vi "运维调试_总磷总氮.vi"() -> ()   [LabVIEW 2016, in "斯坦道总磷总氮.lvlib"]
uses:
  <vilib>/Utility/miscctls.llb/LVPointTypeDef.ctl
  <vilib>/Plasmionique/MB Master/MB_Master/MB_Master.lvclass
  <vilib>/ptbypt/NI_PtbyPt.lvlib
panel:
  out "步骤":u16
  out "seconds since 1Jan1904 2":timestamp
  out "seconds since 1Jan1904":timestamp
  in  "周期设置":bool
  in  "流程操作":bool
  out "消解压力":sgl format="%#.2f kPa"
  out "权限等级":string
  out "总步数":i32
  out "滑动杆":dbl(slide) caption="测试进度" scale=0.0..100.0
  out "试剂余量显示":sgl[][](graph)
  in  "仪器校准":bool
  in  "参数查询":bool
  out "简易步骤名称":string
  in  "温度曲线":bool
  in  "试剂余量":bool
  in  "灯值调整":bool
  out "固件版本号":string
  out "模块版本号":string
  out "注射器温度":sgl format="%#.2f ℃"
  out "消解温度":sgl format="%#.2f ℃"
  out "ADC":sgl
  out "F3":sgl format="%#.6f"
  out "F2":sgl format="%#.6f"
  out "F1":sgl format="%#.6f"
  out "F0":sgl format="%#.6f"
  out "运行状态":T1 {"数据时间:" format="%<%y/%m/%d %H:%M:%S>T"; "仪器时间:" format="%<%y/%m/%d %H:%M:%S>T"}
  in  "单选按钮":T2=enum."总氮"
  in  "布尔":bool
  in  "外设固件":bool
  out "字符串 2":string
  in  "数组":string[](array[string])
  in  "返回":bool
  in  "参数设置":bool
  out "集成报警信息":string
  in  "停止":bool
  in  "手动启动":bool
  in  "调试":bool
  out "多列列表框":i32(listbox)
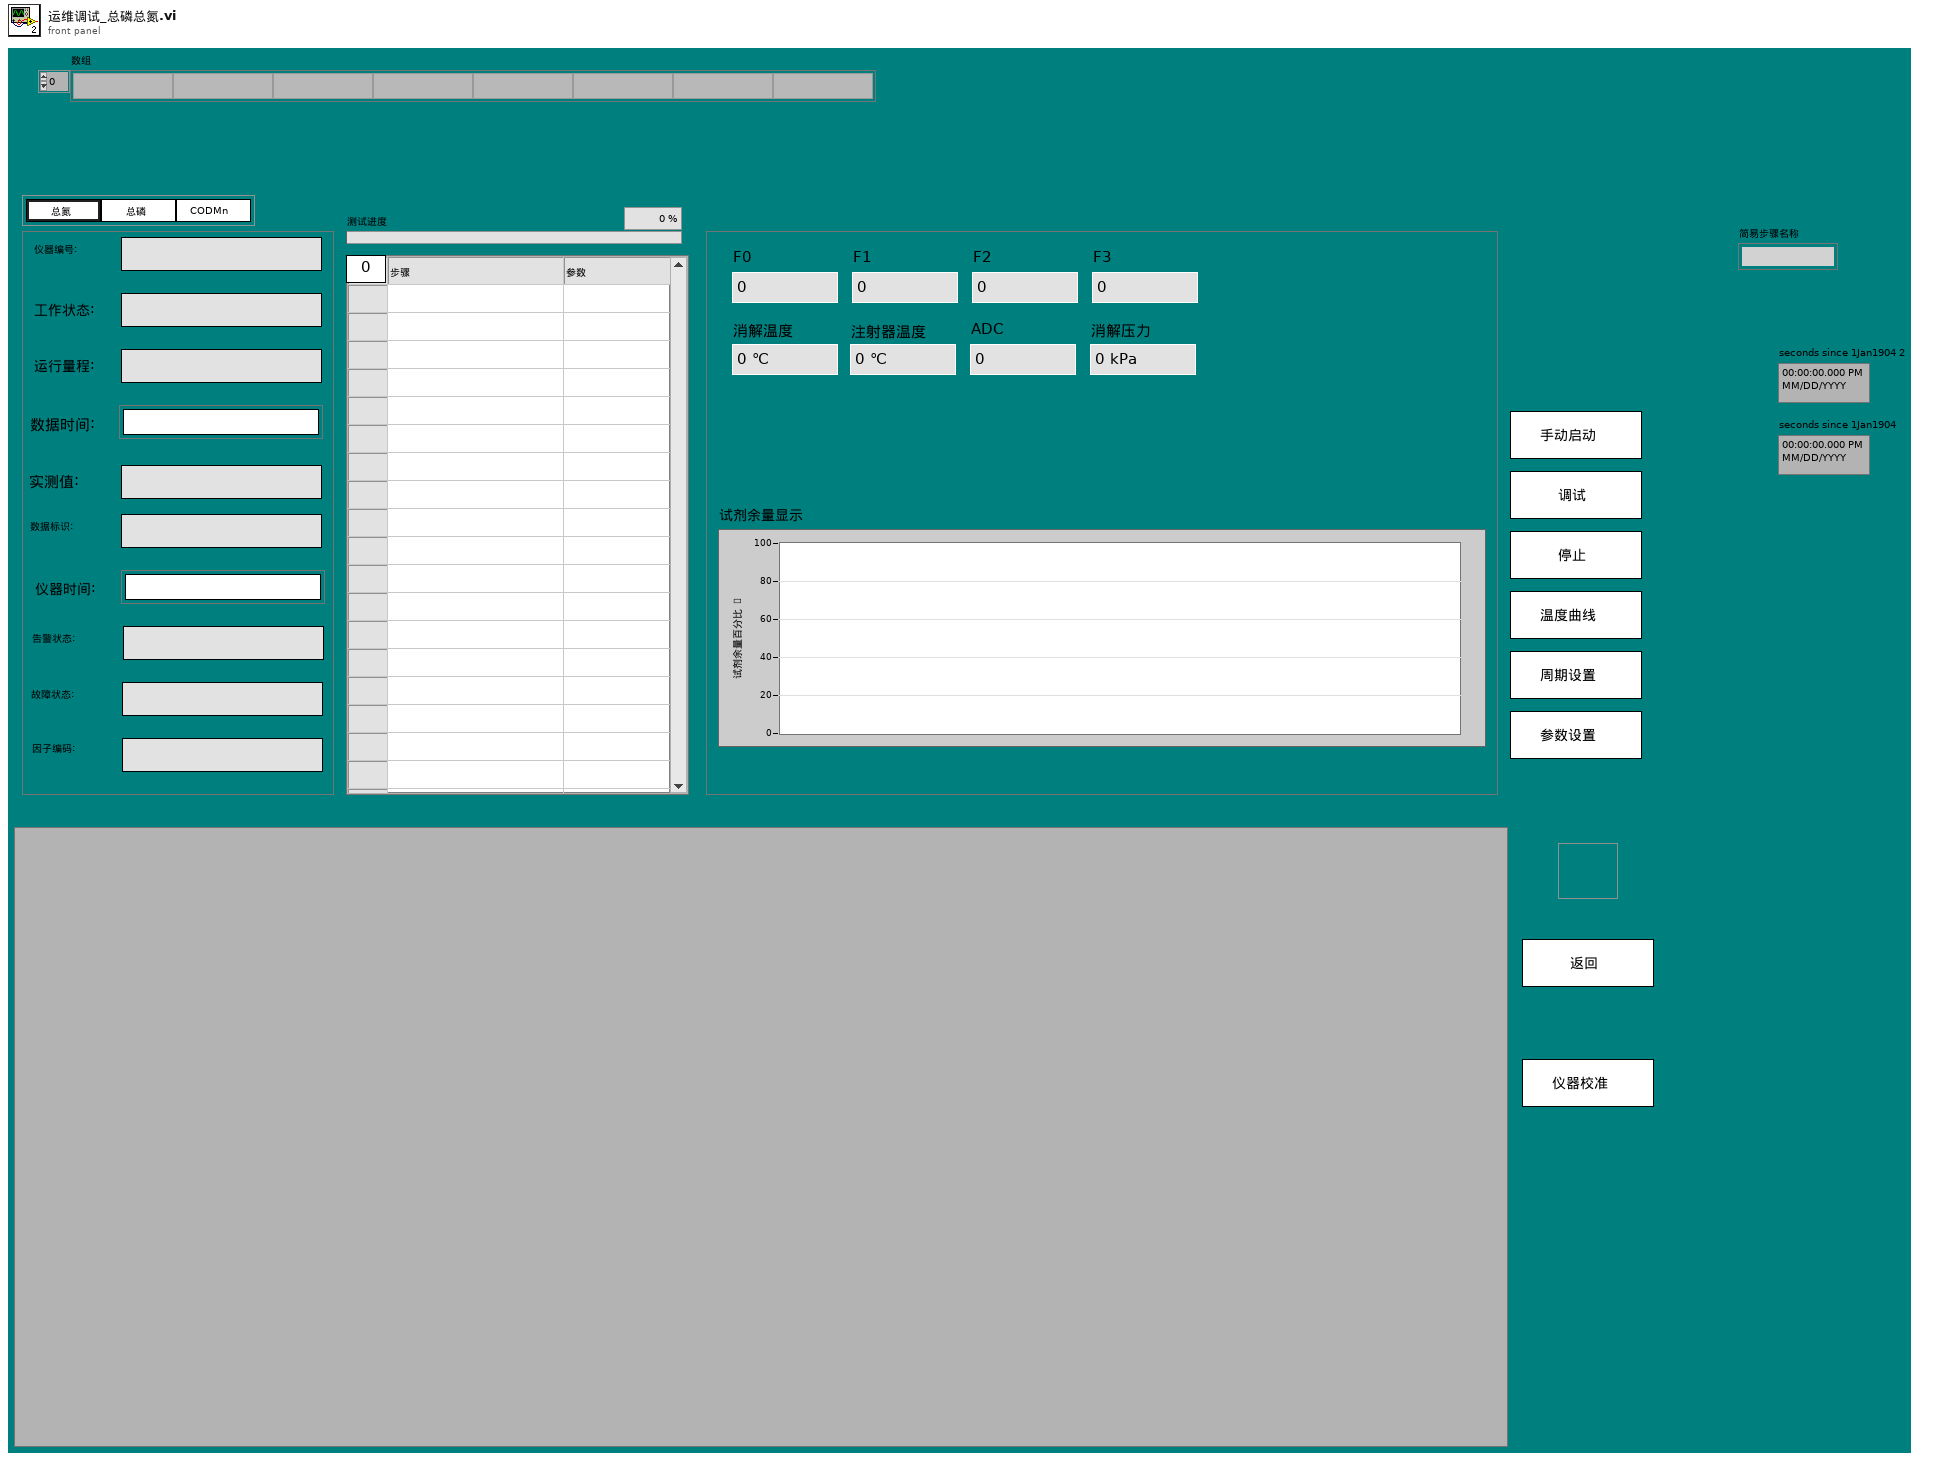
[diagram p1: front panel]
types:
  T1 = cluster{"仪器编号:":string, "工作状态:":string, "运行量程: ":string, "数据时间:":timestamp, "实测值:":string, "数据标识: ":string, "仪器时间:":timestamp, "告警状态: ":string, "故障状态:  ":string, "因子编码:":string}
  T2 = typedef "斯坦道总磷总氮.lvlib/启动参数显示控件.ctl" = enum32{"COD", "氨氮", "总氮", "总磷", "磷酸盐", "硝氮", "亚硝氮", "硅酸盐", "硫化物", "氟化物", "CODMn"}
  T3 = typedef "LVPointTypeDef.ctl" = cluster{"Horizontal":i16, "Vertical":i16}
  T4 = cluster{"系统时间":timestamp, "工作状态":u16, "测量模式":enum16{"待机", "连续模式", "周期模式", "定点模式", "受控模式", "手动模式"}, "告警代码":u16, "故障代码":u16, "日志代码":u16, "软件版本":u16, "F0":sgl, "F1":sgl, "F2":sgl, "F3":sgl, "T":sgl, "H":sgl, "id":u16, "flowid":u16, "量程":u16, "总磷控温温度1":sgl, "营养盐控温温度2":sgl, "ADC":sgl, "结果值":sgl, "运行时间":u16, "步骤详情":string, "步骤流程":string}
  T5 = cluster{"Major":u16, "Minor":u16, "Fix":u16, "Build":u16}
  T6 = typedef "LVStringsAndValuesArrayTypeDef_U16.ctl" = cluster{"String":string, "Value":u16}[]
  T7 = cluster{"因子编码":u32, "单位":u16, "标样参考值":sgl, "水样数据时间":timestamp, "水样实测值":sgl, "水样数据标识":string, "标样数据时间":timestamp, "标样实测值":sgl, "标样数据标识":string, "空白数据时间":timestamp, "空白实测值":sgl, "空白数据标识":string, "零点核查数据时间":timestamp, "零点核查实测值":sgl, "零点核查数据标识":string, "跨度核查数据时间":timestamp, "跨度核查实测值":sgl, "跨度核查数据标识":string, "加标回收数据时间":timestamp, "加标回收实测值":sgl, "加标回收数据标识":string, "平行样数据时间":timestamp, "平行样实测值":sgl, "平行样数据标识":string, "F0":sgl, "F1":sgl, "F2":sgl, "F3":sgl, "F4":sgl, "F5":sgl, "F6":sgl, "F7":sgl, "温度":sgl, "湿度":sgl, "X值":sgl, "fidrange":u16, "X1值":sgl}[]
  T8 = typedef "SingleStepTestV3.lvlib/SingleStepTestV3.lvclass/仪器版本.ctl" = enum16{"V3.1版", "V4版", "V3版", "V4.2版"}
  T9 = cluster{"因子编码":u32, "单位":u16, "标样参考值":sgl, "水样数据时间":timestamp, "水样实测值":sgl, "水样数据标识":string, "标样数据时间":timestamp, "标样实测值":sgl, "标样数据标识":string, "空白数据时间":timestamp, "空白实测值":sgl, "空白数据标识":string, "零点核查数据时间":timestamp, "零点核查实测值":sgl, "零点核查数据标识":string, "跨度核查数据时间":timestamp, "跨度核查实测值":sgl, "跨度核查数据标识":string, "加标回收数据时间":timestamp, "加标回收实测值":sgl, "加标回收数据标识":string, "平行样数据时间":timestamp, "平行样实测值":sgl, "平行样数据标识":string, "F0":sgl, "F1":sgl, "F2":sgl, "F3":sgl, "F4":sgl, "F5":sgl, "F6":sgl, "F7":sgl, "温度":sgl, "湿度":sgl, "X值":sgl, "fidrange":u16, "X1值":sgl}
  T10 = typedef "Alarm interface.lvlib/报警短信语音交互.ctl" = cluster{"参数":string, "元器件":string, "故障现象":string, "code":string, "platform_alarm_code":string, "solutionList":cluster{"reason":string, "solution":string}[], "是否上报":string}
  T11 = typedef "TimingControl.lvlib/TimingControl.lvclass/国标控制命令.ctl" = enum16{"启动测量", "标样核查", "零点核查", "跨度核查", "空白测试", "平行样测试", "加标回收", "空白校准", "标样校准", "初始化（清洗）", "停止测试", "仪器重启", "校时", "模式设置", "测量间隔设置"}
  T12 = typedef "TimingControl.lvlib/TimingControl.lvclass/测量参数.ctl" = u16
  T13 = enum32{"Bad", "Idle", "Run top level", "Running"}
  T14 = cluster{"时间标识":timestamp, "设备":string, "日志信息":string, "流程参数":string}
  T15 = typedef "LVRowAndColumnUnsignedTypeDef.ctl" = cluster{"Row":u32, "Column":u32}
  T16 = typedef "操作日志字段定义.ctl" = cluster{"时间":timestamp, "参数":string, "日志信息":string, "流程参数":string}
  T17 = cluster{"站号":u16, "量程切换":enum32{"H", "L", "AUTO"}, "控制命令":enum16{"启动测量", "标样核查", "零点核查", "跨度核查", "空白测试", "平行样测试", "加标回收", "空白校准", "标样校准", "初始化（清洗）", "停止测试", "仪器重启", "校时", "模式设置", "测量间隔设置"}, "模式设置":enum16{"待机", "连续模式", "周期模式", "定点模式", "受控模式", "手动模式"}, "测量间隔":u16}
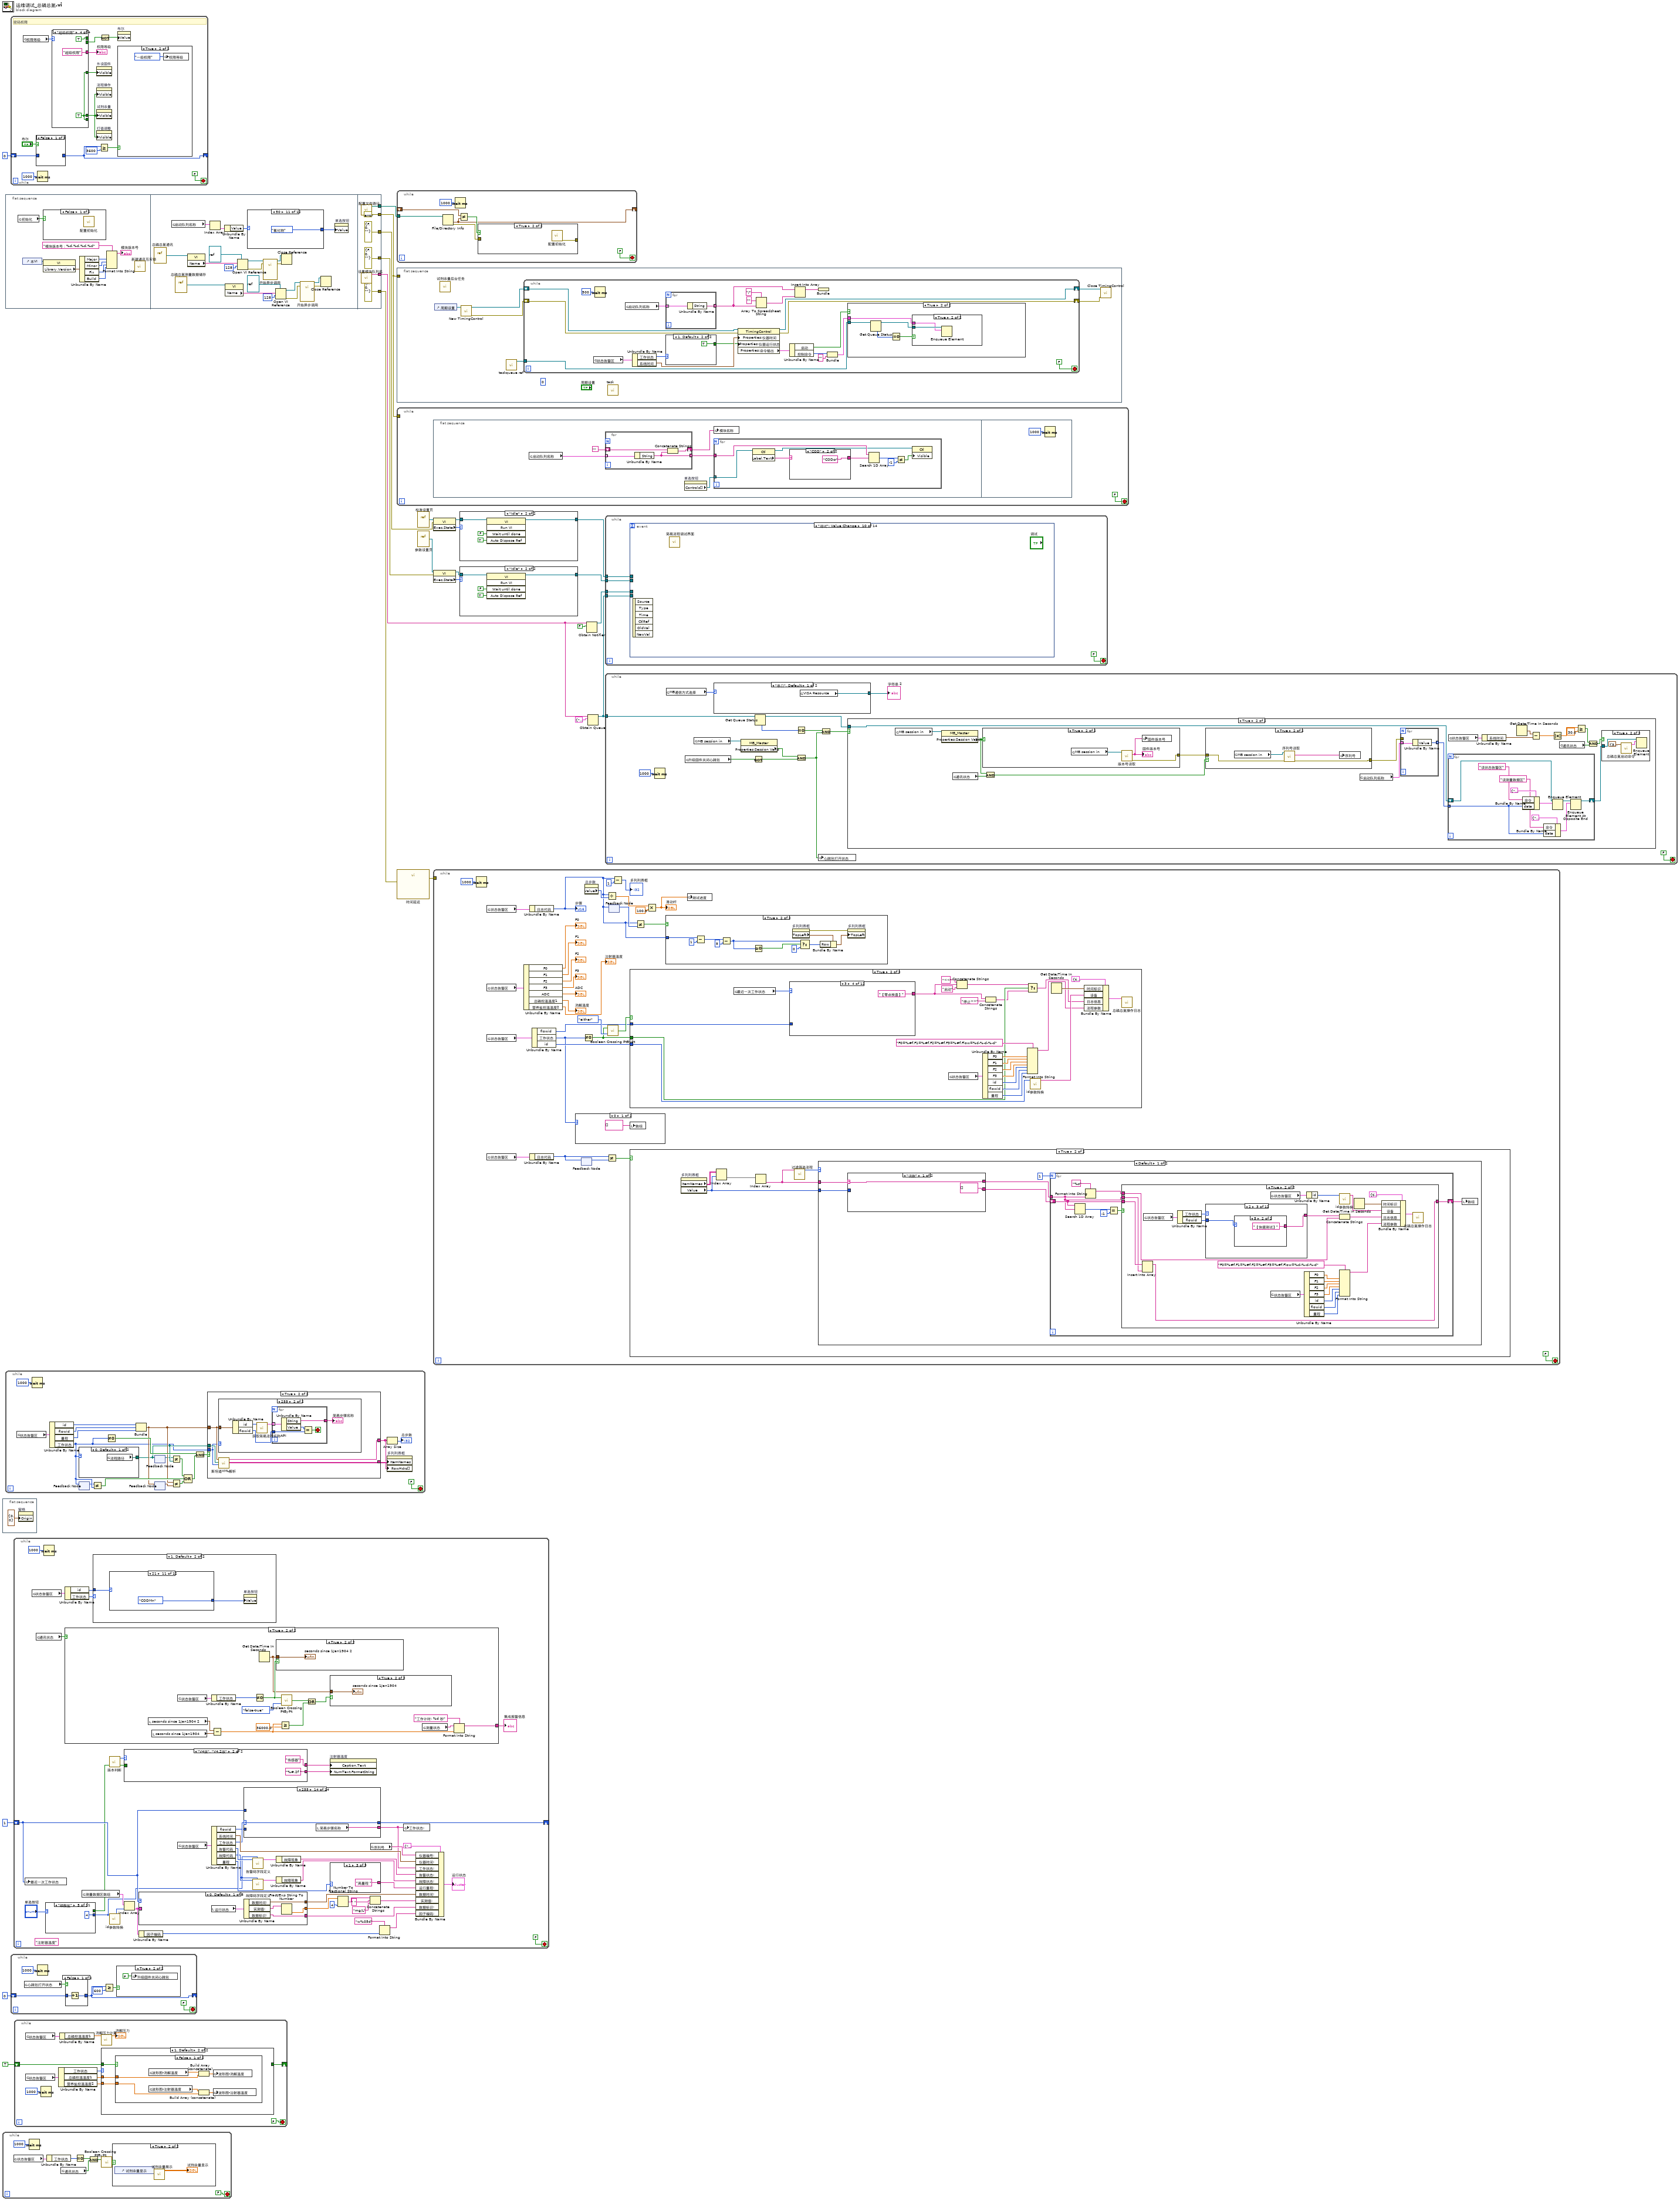
[diagram p0: block diagram]
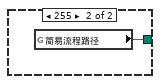
[diagram p2: hidden frame]
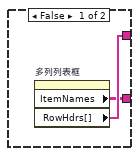
[diagram p3: hidden frame]
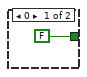
[diagram p7: hidden frame]
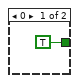
[diagram p14: hidden frame]
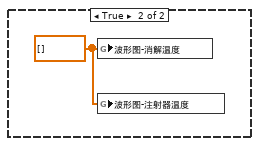
[diagram p15: hidden frame]
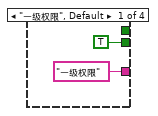
[diagram p17: hidden frame]
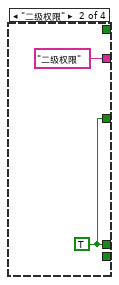
[diagram p18: hidden frame]
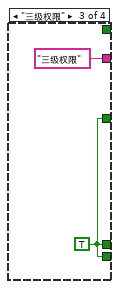
[diagram p19: hidden frame]
diagram:
  n1 = flat-sequence {
    frame #0 {
      n2 = property on="窗格" class="Pane"("Origin"=T3 {"Horizontal"=0, "Vertical"=0} ("原点")) -> ()  [unwired: 2 in, 2 out]
    }
  }
  n3 = while {
    stop <- FALSE stop-if-true
    n4 = global read "VAR总磷总氮全局变量.vi" "状态告警区"() -> (w29:T4)
    n5 = Wait (ms)(milliseconds to wait=u32 1000 ("等待时间（毫秒）")) -> ()  [unwired: 1 out]
    n6 = Unbundle By Name(w29) -> ("工作状态"=w27:u16)
    n7 = global read "VAR总磷总氮全局变量.vi" "通讯状态"() -> (w30:bool)
    n8 = Equal To 0?(x=w27) -> (x = 0?=w26:bool)
    n9 = And(x=w26, y=w30) -> (x .and. y?=w28:bool)
    n10 = call <vilib>:"Boolean Crossing PtByPt.vi"("input"=w28) -> ("crossing"=w25:bool)  [unwired: 2 in]
    n11 = case shown="True" w25 {
      frame False {
      }
      frame True {
        n12 = control-ref of="试剂余量显示"() -> (w33:refnum<vi>)
        n13 = call "试剂余量展示.vi"("波形图 2"=w33) -> ("波形图"=→"试剂余量显示":sgl[][])  [unwired: 10 in]
      }
    }
  }
  n14 = flat-sequence {
    tunnel: [w81] -> w17
    tunnel: [errorcluster {"status"=FALSE, "code"=0, "source"=""} ("错误输入（无错误）")] -> w8
    tunnel: [errorcluster {"status"=FALSE, "code"=0, "source"=""} ("错误输入（无错误）")] -> w7
    tunnel: [w78] -> w5
    tunnel: [errorcluster {"status"=FALSE, "code"=0, "source"=""} ("error out")] -> w4
    tunnel: [errorcluster {"status"=FALSE, "code"=0, "source"=""} ("错误输入（无错误）")] -> w3
    frame #0 {
      n15 = global read "VAR总磷总氮全局变量.vi" "初始化"() -> (w35:bool)
      n16 = control-ref of="本VI"() -> (w43:refnum<vi>)
      n17 = case shown="False" w35 {
        frame False {
          n18 = call "配置初始化.vi"() -> ()  [unwired: 11 in, 1 out]
        }
        frame True {
        }
      }
      n19 = property class="VI"(reference=w43) -> ("Library.Version"=w42:T5)  [unwired: 1 in, 2 out]
      n20 = Unbundle By Name(w42) -> ("Major"=w40:u16, "Minor"=w39:u16, "Fix"=w38:u16, "Build"=w37:u16)
      n21 = Format Into String(format string="模块版本号：%d.%d.%d.%d" ("格式字符串"), w40, w39, w38, w37) -> (resulting string=→"模块版本号":string)  [unwired: 2 in, 1 out]
      n22 = call "新建通讯互斥锁.vi"() -> ()  [unwired: 11 in, 1 out]
    }
    frame #1 {
      n23 = vi-ref "总磷总氮通讯.vi"() -> (w48:refnum<vi>)
      n24 = global read "model config var.vi" "启动队列名称"() -> (w46:cluster{"String":string, "Value":u16}[])
      n25 = vi-ref "总磷总氮测量数据储存.vi"() -> (w56:refnum<vi>)
      n26 = property class="VI"(reference=w48) -> ("Name"=w49:string)  [unwired: 1 in, 2 out]
      n27 = Index Array(array=w46) -> (element=w45:cluster{"String":string, "Value":u16})  [unwired: 1 in]
      n28 = Unbundle By Name(w45) -> ("Value"=w44:u16)
      n29 = property class="VI"(reference=w56) -> ("Name"=w63:string)  [unwired: 1 in, 2 out]
      n30 = Open VI Reference(type specifier VI Refnum (for type only)=refnum<vi> refnum, vi path=w49, options=128 ("选项")) -> (vi reference=w51:refnum<vi>, error out=w53:errorcluster)  [unwired: 3 in]
      n31 = case shown="50" w44 {
        tunnel: [w64 启动参数显示控件."总磷" ("单选按钮") 启动参数显示控件."总氮" ("单选按钮") 启动参数显示控件."COD" ("单选按钮") 启动参数显示控件."氨氮" ("单选按钮") 启动参数显示控件."磷酸盐" ("单选按钮") 启动参数显示控件."硝氮" ("单选按钮") 启动参数显示控件."亚硝氮" ("单选按钮") 启动参数显示控件."硅酸盐" ("单选按钮") 启动参数显示控件."硫化物" ("单选按钮") 启动参数显示控件."氟化物" ("单选按钮") 启动参数显示控件."CODMn" ("单选按钮")] -> w47
        frame 0, Default {
          n32 = property on="单选按钮" class="RadioBtnsControl (strict)"() -> ("Value"=w64:T2)  [unwired: 2 in, 2 out]
        }
        frame 1 {
        }
        frame 2 {
        }
        frame 22 {
        }
        frame 3 {
        }
        frame 4 {
        }
        frame 5 {
        }
        frame 6 {
        }
        frame 7 {
        }
        frame 8 {
        }
        frame 50 {
        }
        frame 21 {
        }
      }
      n33 = call-by-ref "开始异步调用"(reference=w51, error in=w53) -> (reference out=w55:refnum<vi>, error out=w54:errorcluster)  [unwired: 12 in]
      n34 = Open VI Reference(type specifier VI Refnum (for type only)=refnum<vi> refnum, vi path=w63, options=128 ("选项")) -> (vi reference=w61:refnum<vi>, error out=w59:errorcluster)  [unwired: 3 in]
      n35 = Close Reference(reference=w55, error in (no error)=w54) -> ()  [unwired: 1 out]
      n36 = call-by-ref "开始异步调用"(reference=w61, error in=w59) -> (reference out=w57:refnum<vi>, error out=w58:errorcluster)  [unwired: 12 in]
      n37 = Close Reference(reference=w57, error in (no error)=w58) -> ()  [unwired: 1 out]
      n38 = property on="单选按钮" class="RadioBtnsControl (strict)"("Value"=w47) -> ()  [unwired: 2 in, 2 out]
    }
    frame #2 {
      n39 = call "配置文件路径.vi"() -> ("appended path"=w78:path)  [unwired: 11 in]
      n40 = call "设置模块队列名.vi"() -> ("Msg"=w81:string)  [unwired: 5 in]
    }
  }
  n41 = while {
    stop <- FALSE stop-if-true
    n42 = global read "VAR总磷总氮全局变量.vi" "状态告警区"() -> (w93:T4)
    n43 = Wait (ms)(milliseconds to wait=u32 1000 ("等待时间（毫秒）")) -> ()  [unwired: 1 out]
    n44 = Unbundle By Name(w93) -> ("id"=w92:u16, "flowid"=w91:u16, "量程"=w90:u16, "工作状态"=w83:u16)
    n45 = case shown="0, Default" w83 {
      tunnel: [w103 w104] -> w85
      frame 0, Default {
        n46 = global read "总磷总氮断电保存全局变量.vi" "流程路径"() -> (w103:path)
      }
      frame 255 {
        n47 = global read "总磷总氮断电保存全局变量.vi" "简易流程路径"() -> (w104:path)
      }
    }
    n48 = feedback #1() -> (w82:u16)  [unwired: 1 in]
    n49 = feedback-in #1(w83) -> ()
    n50 = Not Equal?(x=w82, y=w83) -> (x != y?=w99:bool)
    n51 = Not Equal To 0?(x=w83) -> (x != 0?=w94:bool)
    n52 = Bundle("id"=w92, "flowid"=w91, "量程"=w90) -> (w87:cluster{"id":u16, "flowid":u16, "量程":u16})  [unwired: 1 in]
    n53 = feedback #2() -> (w84:path)  [unwired: 1 in]
    n54 = feedback-in #2(w85) -> ()
    n55 = feedback-in #3(w87) -> ()
    n56 = feedback #3() -> (w88:cluster{"id":u16, "flowid":u16, "量程":u16})  [unwired: 1 in]
    n57 = Not Equal?(x=w84, y=w85) -> (x != y?=w98:bool)
    n58 = Not Equal?(x=w87, y=w88) -> (x != y?=w86:bool)
    n59 = Compound Arithmetic op=OR ("复合运算")(w98, w99, w86) -> (w100:bool)
    n60 = And(x=w94, y=w100) -> (x .and. y?=w95:bool)
    n61 = case shown="True" w95 {
      tunnel: [w106 w109] -> w97
      tunnel: [w105 w110] -> w101
      tunnel: w87 -> [_ w108]
      tunnel: w85 -> [_ w111]
      tunnel: w83 -> [_ w107]
      frame False {
        n62 = property on="多列列表框" class="MCListbox (strict)"() -> ("ItemNames"=w105:string[][], "RowHdrs[]"=w106:string[])  [unwired: 2 in, 2 out]
      }
      frame True {
        n63 = case shown="255" w107 {
          tunnel: w108 -> [_ w116]
          frame 0, Default {
          }
          frame 255 {
            n64 = Unbundle By Name(w116) -> ("id"=w115:u16, "flowid"=w113:u16)
            n65 = call "获取简易流程名称API.vi"("参数下拉列表"=w115) -> ("字符串与值[]"=w114:T6)  [unwired: 9 in, 1 out]
            n66 = for {
              tunnel: w114 -> [w121] mode=indexing
              tunnel: w113 -> [w119]
              tunnel: [w118] -> w112
              stop <- w117 stop-if-true
              n67 = Unbundle By Name(w121) -> ("String"=w118:string, "Value"=w120:u16)
              n68 = Equal?(x=w120, y=w119) -> (x = y?=w117:bool)
            }
            "简易步骤名称" <- w112
          }
        }
        n69 = call "斯坦道XML解析.vi"("工作状态"=w107, "添加的路径"=w111, "参数簇"=w108) -> ("步骤名"=w110:string[][], "索引"=w109:string[])  [unwired: 6 in, 1 out]
      }
    }
    n70 = Array Size(array=w97) -> (size(s)=→"总步数":i32)
    n71 = property on="多列列表框" class="MCListbox (strict)"("ItemNames"=w101, "RowHdrs[]"=w97) -> ()  [unwired: 2 in, 2 out]
  }
  n72 = while {
    shift-right: [w131] -> _
    shift-left: u32 0 ("y") -> [w133]
    stop <- FALSE stop-if-true
    # "密码权限"
    n73 = global read "VAR总磷总氮全局变量.vi" "权限等级"() -> (w128:enum16{"一级权限", "二级权限", "三级权限", "超级权限"})
    n74 = case shown="False" "布尔" {
      tunnel: w133 -> [_ w146]
      tunnel: [_ w145] -> w131
      frame False {
      }
      frame True {
        n75 = Increment(x=w146) -> (x+1=w145:u32)
      }
    }
    n76 = Wait (ms)(milliseconds to wait=u32 1000 ("等待时间（毫秒）")) -> ()  [unwired: 1 out]
    n77 = case shown="\"超级权限\"" w128 {
      tunnel: [_ w138 w140 w143] -> w122
      tunnel: [_ _ w140 w143] -> _
      tunnel: [_ w138 w140 w143] -> w127
      tunnel: [_ _ _ TRUE] -> _
      tunnel: [TRUE _ _ _] -> w125
      tunnel: ["一级权限" "二级权限" "三级权限" "超级权限"] -> w123
      frame "一级权限", Default {
      }
      frame "二级权限" {
        w138 = TRUE
      }
      frame "三级权限" {
        w140 = TRUE
      }
      frame "超级权限" {
        w143 = TRUE
      }
    }
    "权限等级" <- w123
    n78 = property on="外设固件" class="Bool"("Visible"=w127) -> ()  [unwired: 2 in, 2 out]
    n79 = property on="流程操作" class="Bool"("Visible"=w122) -> ()  [unwired: 2 in, 2 out]
    n80 = property on="试剂余量" class="Bool"("Visible"=w122) -> ()  [unwired: 2 in, 2 out]
    n81 = property on="灯值调整" class="Bool"("Visible"=w122) -> ()  [unwired: 2 in, 2 out]
    n82 = Greater Or Equal?(x=w131, y=u32 3600) -> (x >= y?=w129:bool)
    n83 = Not(x=w125) -> (.not. x?=w124:bool)
    n84 = property on="布尔" class="Bool (strict)"("Value"=w124) -> ()  [unwired: 2 in, 2 out]
    n85 = case shown="True" w129 {
      frame False {
      }
      frame True {
        n86 = global write "VAR总磷总氮全局变量.vi" "权限等级"(enum16{"一级权限", "二级权限", "三级权限", "超级权限"}."一级权限" ("权限等级")) -> ()
      }
    }
  }
  n87 = while {
    shift-right: [w151] -> _
    shift-left: 0 -> [w152]
    stop <- FALSE stop-if-true
    n88 = global read "VAR总磷总氮全局变量.vi" "心跳包打开状态"() -> (w147:bool)
    n89 = Wait (ms)(milliseconds to wait=u32 1000 ("等待时间（毫秒）")) -> ()  [unwired: 1 out]
    n90 = case shown="False" w147 {
      tunnel: w152 -> [w156 _]
      tunnel: [w155 _] -> w151
      frame False {
        n91 = Increment(x=w156) -> (x+1=w155:i32)
      }
      frame True {
      }
    }
    n92 = Greater Or Equal?(x=w151, y=600) -> (x >= y?=w149:bool)
    n93 = case shown="True" w149 {
      frame False {
      }
      frame True {
        n94 = global write "VAR总磷总氮全局变量.vi" "升级固件关闭心跳包"(FALSE ("关闭心跳包")) -> ()
      }
    }
  }
  n95 = while {
    shift-right: [w168] -> _
    shift-left: u16 1 ("工作状态") -> [w166]
    stop <- FALSE stop-if-true
    (unwired) "注射器温度"
    n96 = global write "VAR总磷总氮全局变量.vi" "最近一次工作状态"(w166) -> ()
    n97 = global read "VAR总磷总氮全局变量.vi" "状态告警区"() -> (w188:T4)
    n98 = global read "VAR总磷总氮全局变量.vi" "通讯状态"() -> (w199:bool)
    n99 = Wait (ms)(milliseconds to wait=u32 1000 ("等待时间（毫秒）")) -> ()  [unwired: 1 out]
    n100 = case shown="\"磷酸盐\"" "单选按钮" {
      tunnel: [22 3 2 1 4 5 6 7 8 50 21] -> w157
      tunnel: [_ TRUE _ _ _ _ _ _ _ _ _] -> w160
      frame "COD", Default {
      }
      frame "氨氮" {
      }
      frame "总氮" {
      }
      frame "总磷" {
      }
      frame "磷酸盐" {
      }
      frame "硝氮" {
      }
      frame "亚硝氮" {
      }
      frame "硅酸盐" {
      }
      frame "硫化物" {
      }
      frame "氟化物" {
      }
      frame "CODMn" {
      }
    }
    n101 = Unbundle By Name(w188) -> ("id"=w187:u16, "工作状态"=w183:u16)
    n102 = case shown="True" w199 {
      tunnel: ["通讯异常" ("集成报警信息") w318] -> w198
      frame False {
      }
      frame True {
        n103 = local read "seconds since 1Jan1904 2"() -> (w310:timestamp)
        n104 = local read "seconds since 1Jan1904"() -> (w313:timestamp)
        n105 = global read "VAR总磷总氮全局变量.vi" "状态告警区"() -> (w320:T4)
        n106 = Unbundle By Name(w320) -> ("工作状态"=w316:u16)
        n107 = Subtract(x=w310, y=w313) -> (x-y=w309:dbl)
        n108 = Not Equal To 0?(x=w316) -> (x != 0?=w312:bool)
        n109 = Get Date/Time In Seconds() -> (seconds since 1Jan1904=w311:timestamp)
        n110 = case shown="True" w312 {
          tunnel: w311 -> [_ w321]
          frame False {
          }
          frame True {
            "seconds since 1Jan1904 2" <- w321
          }
        }
        n111 = Greater Or Equal?(x=w309, y=36000.0) -> (x >= y?=w306:bool)
        n112 = call <vilib>:"Boolean Crossing PtByPt.vi"("direction"=enum16{"either", "false-true", "true-false"}."false-true", "input"=w312) -> ("crossing"=w314:bool)  [unwired: 1 in]
        n113 = Or(x=w314, y=w306) -> (x .or. y?=w307:bool)
        n114 = case shown="True" w307 {
          tunnel: w311 -> [_ w322]
          frame False {
          }
          frame True {
            "seconds since 1Jan1904" <- w322
          }
        }
        n115 = global read "VAR总磷总氮全局变量.vi" "测量状态"() -> (w317:string)
        n116 = Format Into String(format string="工作计时: %d 秒" ("格式字符串"), initial string=w317, w309) -> (resulting string=w318:string)  [unwired: 1 in, 1 out]
      }
    }
    "集成报警信息" <- w198
    n117 = global read "VAR总磷总氮全局变量.vi" "测量数据区数组"() -> (w172:T7)
    n118 = case shown="1, Default" w183 {
      tunnel: w187 -> [_ w255]
      frame 0 {
      }
      frame 1, Default {
        n119 = case shown="21" w255 {
          tunnel: [w256 启动参数显示控件."总磷" ("单选按钮") 启动参数显示控件."总氮" ("单选按钮") 启动参数显示控件."COD" ("单选按钮") 启动参数显示控件."氨氮" ("单选按钮") 启动参数显示控件."磷酸盐" ("单选按钮") 启动参数显示控件."硝氮" ("单选按钮") 启动参数显示控件."亚硝氮" ("单选按钮") 启动参数显示控件."硅酸盐" ("单选按钮") 启动参数显示控件."硫化物" ("单选按钮") 启动参数显示控件."CODMn" ("单选按钮") 启动参数显示控件."氟化物" ("单选按钮")] -> w254
          frame 0, Default {
            n120 = property on="单选按钮" class="RadioBtnsControl (strict)"() -> ("Value"=w256:T2)  [unwired: 2 in, 2 out]
          }
          frame 1 {
          }
          frame 2 {
          }
          frame 22 {
          }
          frame 3 {
          }
          frame 4 {
          }
          frame 5 {
          }
          frame 6 {
          }
          frame 7 {
          }
          frame 8 {
          }
          frame 21 {
          }
          frame 50 {
          }
        }
        n121 = property on="单选按钮" class="RadioBtnsControl (strict)"("Value"=w254) -> ()  [unwired: 2 in, 2 out]
      }
    }
    n122 = call "版本判断.vi"() -> ("仪器版本"=w162:T8)  [unwired: 11 in]
    n123 = call "id参数转换.vi"("id"=w157) -> ("数组资源索引"=w169:i32)  [unwired: 9 in, 1 out]
    n124 = case shown="\"V4版\", \"V4.2版\"" w162 {
      tunnel: [w202 "传感器" ("标题.文本")] -> w159
      tunnel: ["%#.2f ℃" ("数值文本.格式字符串") "%#.2f " ("数值文本.格式字符串")] -> w161
      tunnel: w160 -> [w205 _]
      frame "V3.1版", Default {
        n125 = Select(t="显色温度", s=w205, f="注射器温度" ("标题.文本")) -> (s? t:f=w202:string)
      }
      frame "V4版", "V4.2版" {
      }
    }
    n126 = Index Array(array=w172, index=w169) -> (element=w171:T9)
    n127 = case shown="0, Default" w166 {
      tunnel: [w223 w229 w233 w237 w241 w245 w249 w253] -> w182
      tunnel: [w221 w228 w232 w236 w239 w244 w248 w252] -> w177
      tunnel: [w224 w227 w231 w235 w238 w243 w247 w251] -> w175
      tunnel: w171 -> [_ w226 w230 w234 w240 w242 w246 w250]
      frame 0, Default {
        n128 = local read "运行状态"() -> (w225:T1)
        n129 = Unbundle By Name(w225) -> ("数据时间:"=w223:timestamp, "实测值:"=w222:string, "数据标识:"=w224:string)
        n130 = Fract/Exp String To Number(string=w222) -> (number=w221:dbl)  [unwired: 3 in, 1 out]
      }
      frame 1 {
        n131 = Unbundle By Name(w226) -> ("水样数据时间"=w229:timestamp, "水样实测值"=w228:sgl, "水样数据标识"=w227:string)
      }
      frame 2, 9 {
        n132 = Unbundle By Name(w230) -> ("标样数据时间"=w233:timestamp, "标样实测值"=w232:sgl, "标样数据标识"=w231:string)
      }
      frame 3 {
        n133 = Unbundle By Name(w234) -> ("零点核查数据时间"=w237:timestamp, "零点核查实测值"=w236:sgl, "零点核查数据标识"=w235:string)
      }
      frame 4 {
        n134 = Unbundle By Name(w240) -> ("跨度核查数据时间"=w241:timestamp, "跨度核查实测值"=w239:sgl, "跨度核查数据标识"=w238:string)
      }
      frame 7 {
        n135 = Unbundle By Name(w242) -> ("加标回收数据时间"=w245:timestamp, "加标回收实测值"=w244:sgl, "加标回收数据标识"=w243:string)
      }
      frame 5, 8 {
        n136 = Unbundle By Name(w246) -> ("空白数据时间"=w249:timestamp, "空白实测值"=w248:sgl, "空白数据标识"=w247:string)
      }
      frame 6 {
        n137 = Unbundle By Name(w250) -> ("平行样数据时间"=w253:timestamp, "平行样实测值"=w252:sgl, "平行样数据标识"=w251:string)
      }
    }
    n138 = Unbundle By Name(w171) -> ("因子编码"=w173:u32)
    n139 = global read "VAR总磷总氮全局变量.vi" "状态告警区"() -> (w197:T4)
    n140 = Unbundle By Name(w197) -> ("flowid"=w165:u16, "系统时间"=w193:timestamp, "工作状态"=w192:u16, "告警代码"=w186:u16, "故障代码"=w185:u16, "量程"=w191:u16)
    n141 = case shown="255" w192 {
      selector: w192 -> [w272 _ w278 w282 w285 w287 w289 w291 w293 w295 w297 w299 w301 w304]
      tunnel: [w273 "空闲" ("工作状态") "水样测量" ("工作状态") w281 "零点核查" ("工作状态") "跨度核查" ("工作状态") "空白测试" ("工作状态") "平行样测试" ("工作状态") "加标回收" ("工作状态") "空白校准" ("工作状态") "标样校准" ("工作状态") "初始化" ("工作状态") "单步调试" ("工作状态") w303] -> w167
      tunnel: [w271 w276 w278 w282 w285 w287 w289 w291 w293 w295 w297 w299 w301 w304] -> w168
      tunnel: w166 -> [w271 w276 _ _ _ _ _ _ _ _ _ _ _ _]
      tunnel: w165 -> [_ _ _ w280 _ _ _ _ _ _ _ _ _ _]
      frame Default {
        n142 = Format Into String(format string="%d" ("格式字符串"), initial string="未知" ("工作状态"), w272) -> (resulting string=w273:string)  [unwired: 1 in, 1 out]
      }
      frame 0 {
      }
      frame 1 {
      }
      frame 2 {
        n143 = case shown="5" w280 {
          tunnel: ["标样核查" ("工作状态") "快捷测试" ("工作状态")] -> w281
          frame 0, Default {
          }
          frame 5 {
          }
        }
      }
      frame 3 {
      }
      frame 4 {
      }
      frame 5 {
      }
      frame 6 {
      }
      frame 7 {
      }
      frame 8 {
      }
      frame 9 {
      }
      frame 10 {
      }
      frame 254 {
      }
      frame 255 {
        n144 = local read "简易步骤名称"() -> (w303:string)
      }
    }
    n145 = call "告警码字段定义.vi"("id"=w157, "告警代码"=w186) -> ("告警信息"=w164:T10)  [unwired: 9 in]
    n146 = call "故障码字段定义.vi"("id"=w157, "故障代码"=w185) -> ("告警信息"=w184:T10)  [unwired: 9 in]
    n147 = Unbundle By Name(w164) -> ("故障现象"=w163:string)
    n148 = Unbundle By Name(w184) -> ("故障现象"=w158:string)
    n149 = property on="注射器温度" class="DigNum (strict)"("Caption.Text"=w159, "NumText.FormatString"=w161) -> ()  [unwired: 2 in, 2 out]
    n150 = case shown="1" w191 {
      tunnel: ["" ("字符串") "低量程 " ("字符串") "高量程 " ("字符串")] -> w190
      frame Default {
      }
      frame 0 {
      }
      frame 1 {
      }
    }
    n151 = Number To Fractional String(number=w177, precision (6)=i16 4 ("精度(6)")) -> (F-format string=w179:string)  [unwired: 2 in]
    n152 = Concatenate Strings(w179, " " ("字符串"), "mg/L" ("字符串")) -> (w176:string)
    n153 = global read "VAR总磷总氮全局变量.vi" "序列号"() -> (w194:string)
    n154 = Format Into String(format string="w%05d" ("格式字符串"), w173) -> (resulting string=w189:string)  [unwired: 2 in, 1 out]
    n155 = global write "VAR总磷总氮全局变量.vi" "工作状态:"(w167) -> ()
    n156 = Bundle By Name(cluster=T1 {"仪器编号:"="", "工作状态:"="", "运行量程: "="", "数据时间:"=timestamp(0 s since 1904-01-01), "实测值:"="", "数据标识: "="", "仪器时间:"=timestamp(0 s since 1904-01-01), "告警状态: "="", "故障状态:  "="", "因子编码:"=""} ("运行状态"), "仪器编号:"=w194, "仪器时间:"=w193, "工作状态:"=w167, "告警状态:"=w163, "故障状态:"=w158, "运行量程:"=w190, "数据时间:"=w182, "实测值:"=w176, "数据标识:"=w175, "因子编码:"=w189) -> (→"运行状态":T1)
  }
  n157 = while {
    shift-right: [w324] -> _
    shift-left: TRUE -> [w325]
    stop <- FALSE stop-if-true
    n158 = global read "VAR总磷总氮全局变量.vi" "状态告警区"() -> (w328:T4)
    n159 = global read "VAR总磷总氮全局变量.vi" "状态告警区"() -> (w331:T4)
    n160 = Wait (ms)(milliseconds to wait=u32 1000 ("等待时间（毫秒）")) -> ()  [unwired: 1 out]
    n161 = Unbundle By Name(w331) -> ("工作状态"=w326:u16, "总磷控温温度1"=w330:sgl, "营养盐控温温度2"=w329:sgl)
    n162 = Unbundle By Name(w328) -> ("总磷控温温度1"=w327:sgl)
    n163 = call "消解压力计算.vi"("当前消解温度"=w327) -> ("消解压力"=→"消解压力":dbl)  [unwired: 10 in]
    n164 = case shown="1, Default" w326 {
      tunnel: w330 -> [_ w337]
      tunnel: w329 -> [_ w336]
      tunnel: w325 -> [_ w335]
      tunnel: [TRUE _] -> w324
      frame 0 {
      }
      frame 1, Default {
        n165 = case shown="False" w335 {
          tunnel: w337 -> [w343 _]
          tunnel: w336 -> [w342 _]
          frame False {
            n166 = global read "VAR总磷总氮全局变量.vi" "波形图-消解温度"() -> (w341:sgl[])
            n167 = global read "VAR总磷总氮全局变量.vi" "波形图-注射器温度"() -> (w340:sgl[])
            n168 = Build Array (concatenate)(w341, w343) -> (w339:sgl[])
            n169 = Build Array (concatenate)(w340, w342) -> (w338:sgl[])
            n170 = global write "VAR总磷总氮全局变量.vi" "波形图-消解温度"(w339) -> ()
            n171 = global write "VAR总磷总氮全局变量.vi" "波形图-注射器温度"(w338) -> ()
          }
          frame True {
            w344 = dbl[] [] ("波形图-消解温度")
            n172 = global write "VAR总磷总氮全局变量.vi" "波形图-消解温度"(w344) -> ()
            n173 = global write "VAR总磷总氮全局变量.vi" "波形图-注射器温度"(w344) -> ()
          }
        }
      }
    }
  }
  n174 = while {
    shift-right: [w345] -> _
    shift-left: _ -> [w350]
    tunnel: w5 -> [w348]
    stop <- FALSE stop-if-true
    n175 = File/Directory Info(path=w348) -> (last mod=w345:timestamp, error out=w346:errorcluster)  [unwired: 1 in, 5 out]
    n176 = Wait (ms)(milliseconds to wait=u32 1000 ("等待时间（毫秒）")) -> ()  [unwired: 1 out]
    n177 = Not Equal?(x=w350, y=w345) -> (x != y?=w349:bool)
    n178 = case shown="True" w349 {
      tunnel: [_ w352] -> _
      tunnel: w346 -> [_ _]
      frame False {
      }
      frame True {
        n179 = call "配置初始化.vi"() -> ("error out"=w352:errorcluster)  [unwired: 11 in]
      }
    }
  }
  n180 = flat-sequence {
    tunnel: w4 -> [_]
    frame #0 {
      (unwired) u32 0 ("等待时间（毫秒）")
      n181 = control-ref of="周期设置"() -> (w357:refnum<vi>)
      n182 = call "试剂余量后台任务.vi"() -> ()  [unwired: 12 in]
      n183 = call "New TimingControl.vi"("Reference"=w357) -> ("error out"=w355:errorcluster, "TimingControl out"=w356:refnum<class "TimingControl.lvclass">)  [unwired: 9 in]
      n184 = call "taskqueue ref.vi"() -> ("队列输出"=w358:refnum<queue>)  [unwired: 10 in, 1 out]
      n185 = while {
        tunnel: w358 -> [w377]
        shift-right: [w370] -> w354
        shift-left: w356 -> [w375]
        shift-right: [w369] -> w353
        shift-left: w355 -> [w374]
        stop <- FALSE stop-if-true
        n186 = global read "VAR总磷总氮全局变量.vi" "状态告警区"() -> (w378:T4)
        n187 = Wait (ms)(milliseconds to wait=u32 500 ("等待时间（毫秒）")) -> ()  [unwired: 1 out]
        n188 = global read "model config var.vi" "启动队列名称"() -> (w364:cluster{"String":string, "Value":u16}[])
        n189 = Unbundle By Name(w378) -> ("工作状态"=w376:u16, "系统时间"=w372:timestamp)
        n190 = for {
          tunnel: w364 -> [w389] mode=indexing
          tunnel: [w388] -> w363 mode=indexing
          n191 = Unbundle By Name(w389) -> ("String"=w388:string)
        }
        n192 = case shown="1, Default" w376 {
          tunnel: [FALSE TRUE] -> w371
          frame 0 {
          }
          frame 1, Default {
          }
        }
        n193 = property class="TimingControl"(reference=w375, error in=w374, "Properties:仪器时间"=w372, "Properties:仪器运行状态"=w371) -> (reference out=w370:refnum<class "TimingControl.lvclass">, error out=w369:errorcluster, "Properties:命令输出"=w373:cluster{"启动":bool, "控制命令":T11, "测量参数":T12})
        n194 = Array To Spreadsheet String(delimiter (Tab)="/" ("分隔符(Tab)"), array=w363, 3:"" ("格式字符串")) -> (spreadsheet string=w366:string)
        n195 = Unbundle By Name(w373) -> ("启动"=w360:bool, "控制命令"=w362:T11)
        n196 = Insert Into Array(array=w363, new element=w366) -> (w365:string[])  [unwired: 1 in]
        n197 = Bundle(w365) -> ()  [unwired: 1 in, 1 out]
        n198 = Bundle("控制命令"=w362, "") -> (w361:cluster{"控制命令":T11, string})  [unwired: 1 in]
        n199 = case shown="True" w360 {
          tunnel: w361 -> [_ w382]
          tunnel: w377 -> [_ w385]
          frame False {
          }
          frame True {
            n200 = Get Queue Status(queue=w385) -> (queue out=w383:refnum<queue>, # elements in queue=w384:i32)  [unwired: 2 in, 6 out]
            n201 = Equal To 0?(x=w384) -> (x = 0?=w381:bool)
            n202 = case shown="True" w381 {
              tunnel: w383 -> [_ w387]
              tunnel: w382 -> [_ w386]
              frame False {
              }
              frame True {
                n203 = Enqueue Element(queue=w387, element=w386) -> ()  [unwired: 2 in, 3 out]
              }
            }
          }
        }
      }
      n204 = call "task.vi"() -> ()  [unwired: 12 in]
      n205 = call "Close TimingControl.vi"("error in (no error)"=w353, "TimingControl in"=w354) -> ()  [unwired: 9 in, 1 out]
    }
  }
  n206 = while {
    tunnel: w4 -> [_]
    stop <- FALSE stop-if-true
    n207 = flat-sequence {
      frame #0 {
        n208 = global read "model config var.vi" "启动队列名称"() -> (w393:cluster{"String":string, "Value":u16}[])
        n209 = for {
          tunnel: w393 -> [w401] mode=indexing
          shift-right: [w400] -> w396
          shift-left: "" -> [w399]
          tunnel: [w398] -> w394 mode=indexing
          n210 = Unbundle By Name(w401) -> ("String"=w398:string)
          n211 = Concatenate Strings(w399, w398) -> (w400:string)
        }
        n212 = property on="单选按钮" class="RadioBtnsControl (strict)"() -> ("Controls[]"=w395:refnum<vi>[])  [unwired: 2 in, 2 out]
        n213 = global write "VAR总磷总氮全局变量.vi" "模块名称"(w396) -> ()
        n214 = for {
          tunnel: w395 -> [w409] mode=indexing
          tunnel: w394 -> [w408]
          n215 = property class="Ctl"(reference=w409) -> (reference out=w407:refnum<vi>, "Label.Text"=w403:string)  [unwired: 1 in, 1 out]
          n216 = case shown="\"COD\"" w403 {
            selector: w403 -> [w410 _]
            tunnel: [w410 "CODcr"] -> w402
            frame Default {
            }
            frame "COD" {
            }
          }
          n217 = Search 1D Array(1D array=w408, element=w402) -> (index of element=w406:i32)  [unwired: 1 in]
          n218 = Not Equal?(x=w406, y=-1) -> (x != y?=w404:bool)
          n219 = property class="Ctl"(reference=w407, "Visible"=w404) -> ()  [unwired: 1 in, 2 out]
        }
      }
      frame #1 {
        n220 = Wait (ms)(milliseconds to wait=u32 1000 ("等待时间（毫秒）")) -> ()  [unwired: 1 out]
      }
    }
  }
  n221 = call "时间延迟"("error in (no error)"=w3) -> ("error out"=w23:errorcluster)  [unwired: 10 in]
  n222 = vi-ref "校准设置页.vi"() -> (w12:refnum<vi>)
  n223 = vi-ref "参数设置页.vi"() -> (w16:refnum<vi>)
  n224 = property class="VI"(reference=w12, error in=w7) -> (reference out=w10:refnum<vi>, "Exec.State"=w11:T13)  [unwired: 1 out]
  n225 = property class="VI"(reference=w16, error in=w8) -> (reference out=w14:refnum<vi>, "Exec.State"=w15:T13)  [unwired: 1 out]
  n226 = while {
    tunnel: w23 -> [_]
    stop <- FALSE stop-if-true
    n227 = Wait (ms)(milliseconds to wait=u32 1000 ("等待时间（毫秒）")) -> ()  [unwired: 1 out]
    n228 = global read "VAR总磷总氮全局变量.vi" "状态告警区"() -> (w438:T4)
    n229 = global read "VAR总磷总氮全局变量.vi" "状态告警区"() -> (w439:T4)
    n230 = global read "VAR总磷总氮全局变量.vi" "状态告警区"() -> (w437:T4)
    n231 = global read "VAR总磷总氮全局变量.vi" "状态告警区"() -> (w435:T4)
    n232 = Unbundle By Name(w439) -> ("F0"=→"F0":sgl, "F1"=→"F1":sgl, "F2"=→"F2":sgl, "F3"=→"F3":sgl, "ADC"=→"ADC":sgl, "总磷控温温度1"=→"消解温度":sgl, "营养盐控温温度2"=→"注射器温度":sgl)
    n233 = Unbundle By Name(w438) -> ("日志代码"=w413:u16)
    "步骤" <- w413
    n234 = Unbundle By Name(w435) -> ("日志代码"=w434:u16)
    n235 = Unbundle By Name(w437) -> ("flowid"=w417:u16, "工作状态"=w430:u16, "id"=w431:u16)
    n236 = case shown="0" w430 {
      frame 0 {
        n237 = local write "数组"(string[] [] ("数组")) -> ()
      }
      frame 1, Default {
      }
    }
    n238 = feedback #4() -> (w436:u16)  [unwired: 1 in]
    n239 = feedback-in #4(w434) -> ()
    n240 = Not Equal To 0?(x=w430) -> (x != 0?=w415:bool)
    n241 = property on="总步数" class="DigNum (strict)"() -> ("Value"=w420:i32)  [unwired: 2 in, 2 out]
    n242 = Divide(x=w413, y=w420) -> (x/y=w419:dbl)
    n243 = Not Equal?(x=w434, y=w436) -> (x != y?=w433:bool)
    n244 = call <vilib>:"Boolean Crossing PtByPt.vi"("direction"=enum16{"either", "false-true", "true-false"}."either", "input"=w415) -> ("crossing"=w428:bool)  [unwired: 1 in]
    n245 = feedback-in #5(w413) -> ()
    n246 = feedback #5() -> (w441:u16)  [unwired: 1 in]
    n247 = Subtract(x=w413, y=1) -> (x-y=→"多列列表框":i32)
    n248 = case shown="True" w428 {
      tunnel: w431 -> [_ w464]
      tunnel: w417 -> [_ w452]
      tunnel: w415 -> [_ w450]
      frame False {
      }
      frame True {
        n249 = global read "VAR总磷总氮全局变量.vi" "最近一次工作状态"() -> (w451:u16)
        n250 = case shown="3" w451 {
          selector: w451 -> [w470 _ _ _ _ _ _ _ _ _ _ _]
          tunnel: [w469 "【水样测试】" ("字符串") w473 "【零点核查】" ("字符串") "【跨度核查】" ("字符串") "【空白测试】" ("字符串") "【平行样测试】" ("字符串") "【加标回收】" ("字符串") "【空白校准】" ("字符串") "【标样校准】" ("字符串") "【单步调试】" ("字符串") "【简易流程】" ("字符串")] -> w445
          tunnel: w452 -> [_ _ w472 _ _ _ _ _ _ _ _ _]
          frame 0, Default {
            n251 = Number To Decimal String(number=w470) -> (decimal integer string=w469:string)  [unwired: 1 in]
          }
          frame 1 {
          }
          frame 2 {
            n252 = case shown="0, Default" w472 {
              tunnel: ["【标样核查】" ("字符串") "【快捷测试】" ("字符串")] -> w473
              frame 0, Default {
              }
              frame 5 {
              }
            }
          }
          frame 3 {
          }
          frame 4 {
          }
          frame 5 {
          }
          frame 6 {
          }
          frame 7 {
          }
          frame 8 {
          }
          frame 9 {
          }
          frame 254 {
          }
          frame 255 {
          }
        }
        n253 = global read "VAR总磷总氮全局变量.vi" "状态告警区"() -> (w462:T4)
        n254 = Concatenate Strings("<<" ("字符串"), w445, "启动" ("字符串")) -> (w444:string)
        n255 = Unbundle By Name(w462) -> ("F0"=w461:sgl, "F1"=w460:sgl, "F2"=w459:sgl, "F3"=w458:sgl, "id"=w457:u16, "flowid"=w456:u16, "量程"=w455:u16)
        n256 = Concatenate Strings(w445, "停止>>" ("字符串")) -> (w448:string)
        n257 = Format Into String(format string="F0=%#f,F1=%#f,F2=%#f,F3=%#f,Flow=%d-%-d-%-d" ("格式字符串"), w461, w460, w459, w458, w457, w456, w455) -> (resulting string=w453:string)  [unwired: 2 in, 1 out]
        n258 = Select(t=w444, s=w450, f=w448) -> (s? t:f=w449:string)
        n259 = call "id参数转换.vi"("id"=w464) -> ("table输出"=w463:string)  [unwired: 9 in, 1 out]
        n260 = Get Date/Time In Seconds() -> (seconds since 1Jan1904=w467:timestamp)
        n261 = Bundle By Name(cluster=T14 {"时间标识"=timestamp(0 s since 1904-01-01), "设备"="", "日志信息"="", "流程参数"=""} ("data in"), "时间标识"=w467, "设备"=w463, "日志信息"=w449, "流程参数"=w453) -> (w466:T14)
        n262 = call "总磷总氮操作日志.vi"("data in"=w466) -> ()  [unwired: 10 in, 1 out]
      }
    }
    n263 = case shown="True" w433 {
      frame False {
      }
      frame True {
        n264 = property on="多列列表框" class="MCListbox (strict)"() -> ("ItemNames"=w490:string[][], "Value"=w486:i32)  [unwired: 2 in, 2 out]
        n265 = Index Array(array=w490, index (row)=w486) -> (element=w489:string[])  [unwired: 1 in]
        n266 = Index Array(array=w489) -> (element=w488:string)  [unwired: 1 in]
        n267 = call "过滤筛选流程.vi"("字符串"=w488) -> ("匹配后偏移量"=w487:i32)  [unwired: 10 in]
        n268 = case shown="Default" w487 {
          tunnel: w488 -> [w492 _]
          tunnel: w486 -> [w491 _]
          frame Default {
            n269 = case shown="\"读数\"" w492 {
              selector: w492 -> [w498 w505]
              tunnel: [w498 w505] -> w494
              tunnel: [string[] [] ("数组") w500] -> w493
              tunnel: w491 -> [_ w504]
              frame "读数" {
              }
              frame Default {
                n270 = Equal?(x=w504, y=1) -> (x = y?=w502:bool)
                n271 = Select(t=string[] [], s=w502, f="数组") -> (s? t:f=w500:string[])
              }
            }
            n272 = for {
              N: 1 -> [_]
              tunnel: w494 -> [w507]
              shift-right: [w506] -> w495
              shift-left: w493 -> [w508]
              n273 = Search 1D Array(1D array=w508, element=w507) -> (index of element=w511:i32)  [unwired: 1 in]
              n274 = Format Into String(format string="%s" ("格式字符串"), w507) -> (resulting string=w512:string)  [unwired: 2 in, 1 out]
              n275 = Equal?(x=w511, y=-1) -> (x = y?=w509:bool)
              n276 = case shown="True" w509 {
                tunnel: w512 -> [_ w522]
                tunnel: w508 -> [w514 w526]
                tunnel: w507 -> [_ w525]
                tunnel: [w514 w524] -> w506
                frame False {
                }
                frame True {
                  n277 = Insert Into Array(array=w526, new element=w525) -> (w524:string[])  [unwired: 1 in]
                  n278 = global read "VAR总磷总氮全局变量.vi" "状态告警区"() -> (w521:T4)
                  n279 = Unbundle By Name(w521) -> ("工作状态"=w520:u16, "flowid"=w515:u16)
                  n280 = case shown="2" w520 {
                    selector: w520 -> [w541 _ _ _ _ _ _ _ _ _ _ _]
                    tunnel: [w540 "【水样测试】" ("字符串") w544 "【零点核查】" ("字符串") "【跨度核查】" ("字符串") "【空白测试】" ("字符串") "【平行样测试】" ("字符串") "【加标回收】" ("字符串") "【空白校准】" ("字符串") "【标样校准】" ("字符串") "【单步调试】" ("字符串") w555] -> w518
                    tunnel: w515 -> [_ _ w543 _ _ _ _ _ _ _ _ _]
                    frame 0, Default {
                      n281 = Number To Decimal String(number=w541) -> (decimal integer string=w540:string)  [unwired: 1 in]
                    }
                    frame 1 {
                    }
                    frame 2 {
                      n282 = case shown="5" w543 {
                        tunnel: ["【标样核查】" ("字符串") "【快捷测试】" ("字符串")] -> w544
                        frame Default {
                        }
                        frame 5 {
                        }
                      }
                    }
                    frame 3 {
                    }
                    frame 4 {
                    }
                    frame 5 {
                    }
                    frame 6 {
                    }
                    frame 7 {
                    }
                    frame 8 {
                    }
                    frame 9 {
                    }
                    frame 254 {
                    }
                    frame 255 {
                      n283 = local read "简易步骤名称"() -> (w557:string)
                      n284 = Format Into String(format string="(%s)" ("格式字符串"), initial string="【简易流程】" ("工作状态"), w557) -> (resulting string=w555:string)  [unwired: 1 in, 1 out]
                    }
                  }
                  n285 = global read "VAR总磷总氮全局变量.vi" "状态告警区"() -> (w539:T4)
                  n286 = global read "VAR总磷总氮全局变量.vi" "状态告警区"() -> (w536:T4)
                  n287 = Unbundle By Name(w536) -> ("F0"=w533:sgl, "F1"=w532:sgl, "F2"=w531:sgl, "F3"=w530:sgl, "id"=w529:u16, "flowid"=w528:u16, "量程"=w527:u16)
                  n288 = Unbundle By Name(w539) -> ("id"=w517:u16)
                  n289 = call "id参数转换.vi"("id"=w517) -> ("table输出"=w516:string)  [unwired: 9 in, 1 out]
                  n290 = Concatenate Strings(w518, w522) -> (w519:string)
                  n291 = Format Into String(format string="F0=%#f,F1=%#f,F2=%#f,F3=%#f,Flow=%d-%-d-%-d" ("格式字符串"), w533, w532, w531, w530, w529, w528, w527) -> (resulting string=w534:string)  [unwired: 2 in, 1 out]
                  n292 = Get Date/Time In Seconds() -> (seconds since 1Jan1904=w537:timestamp)
                  n293 = Bundle By Name(cluster=T14 {"时间标识"=timestamp(0 s since 1904-01-01), "设备"="", "日志信息"="", "流程参数"=""} ("data in"), "时间标识"=w537, "设备"=w516, "日志信息"=w519, "流程参数"=w534) -> (w538:T14)
                  n294 = call "总磷总氮操作日志.vi"("data in"=w538) -> ()  [unwired: 10 in, 1 out]
                }
              }
            }
            n295 = local write "数组"(w495) -> ()
          }
          frame -1 {
          }
        }
      }
    }
    n296 = Not Equal?(x=w413, y=w441) -> (x != y?=w440:bool)
    n297 = Multiply(x=w419, y=100.0) -> (x*y=w416:dbl)
    "滑动杆" <- w416
    n298 = case shown="True" w440 {
      tunnel: w413 -> [_ w561]
      frame False {
      }
      frame True {
        n299 = Subtract(x=w561, y=1) -> (x-y=w559:i32)
        n300 = Subtract(x=w559, y=5) -> (x-y=w563:i32)
        n301 = Greater Or Equal To 0?(x=w563) -> (x >= 0?=w562:bool)
        n302 = property on="多列列表框" class="MCListbox (strict)"() -> (error out=w567:errorcluster, "TopLeft"=w568:T15)  [unwired: 2 in, 1 out]
        n303 = Select(t=w563, s=w562, f=0) -> (s? t:f=w564:i32)
        n304 = Bundle By Name(cluster=w568, "Row"=w564) -> (w569:T15)
        n305 = property on="多列列表框" class="MCListbox (strict)"(error in=w567, "TopLeft"=w569) -> ()  [unwired: 1 in, 2 out]
      }
    }
    n306 = global write "VAR总磷总氮全局变量.vi" "测试进度"(w416) -> ()
  }
  n307 = case shown="\"Idle\"" w11 {
    tunnel: w10 -> [w570 w574]
    tunnel: [w570 w571] -> w9
    frame "Bad", Default {
    }
    frame "Idle" {
      n308 = invoke class="VI" method="Run VI"(reference=w574, "Wait until done"=FALSE ("结束前等待"), "Auto Dispose Ref"=TRUE ("自动销毁引用")) -> (reference out=w571:refnum<vi>)  [unwired: 2 in, 4 out]
    }
  }
  n309 = case shown="\"Idle\"" w15 {
    tunnel: w14 -> [w575 w579]
    tunnel: [w575 w576] -> w13
    frame "Bad", Default {
    }
    frame "Idle" {
      n310 = invoke class="VI" method="Run VI"(reference=w579, "Wait until done"=FALSE ("结束前等待"), "Auto Dispose Ref"=TRUE ("自动销毁引用")) -> (reference out=w576:refnum<vi>)  [unwired: 2 in, 4 out]
    }
  }
  n311 = Obtain Notifier(name (unnamed)=w17, notification data type=FALSE) -> (notifier out=w18:refnum<notifier>)  [unwired: 2 in, 2 out]
  n312 = Obtain Queue(name (unnamed)=w17, element data type=cluster{"命令":string, "data":variant} {"命令"="", "data"=variant}) -> (queue out=w20:refnum<queue>)  [unwired: 3 in, 2 out]
  n313 = while {
    tunnel: w20 -> [w583]
    tunnel: w18 -> [w582]
    tunnel: w13 -> [w581]
    tunnel: w9 -> [w580]
    stop <- FALSE stop-if-true
    n314 = event shown="[9] \"调试\": Value Change" {
      selector: _ -> [_ _ _ _ _ _ _ _ _ _ _ _ _ _]
      dyn-events: _ -> [_ _ _ _ _ _ _ _ _ _ _ _ _ _]
      timeout: _ -> [_ _ _ _ _ _ _ _ _ _ _ _ _ _]
      tunnel: w583 -> [_ _ _ _ _ _ _ _ w597 _ w604 _ _ _]
      tunnel: w582 -> [_ _ _ _ _ _ _ _ _ _ w603 _ _ _]
      tunnel: w581 -> [_ _ _ _ _ _ _ _ _ _ _ w624 _ _]
      tunnel: w580 -> [_ _ _ _ _ _ _ _ _ _ _ _ w630 _]
      event Timeout {
        n315 = event-data() -> ()  [unwired: 1 in, 3 out]
      }
      event "流程操作": Value Change {
        n316 = event-data() -> ()  [unwired: 1 in, 6 out]
        n317 = global read "总磷总氮断电保存全局变量.vi" "简易流程路径"() -> (w585:path)
        n318 = global read "总磷总氮断电保存全局变量.vi" "流程路径"() -> (w586:path)
        n319 = call "流程批量写入.vi"("简易流程路径"=w585, "添加的路径"=w586) -> ()  [unwired: 10 in]
      }
      event "温度曲线": Value Change {
        n320 = event-data() -> ()  [unwired: 1 in, 6 out]
        n321 = call "温度曲线显示.vi"() -> ()  [unwired: 12 in]
      }
      event "试剂余量": Value Change {
        n322 = event-data() -> ()  [unwired: 1 in, 6 out]
        n323 = call "试剂余量显示UI.vi"() -> ()  [unwired: 12 in]
      }
      event "灯值调整": Value Change {
        n324 = event-data() -> ()  [unwired: 1 in, 6 out]
        n325 = call "灯值调整对话框.vi"() -> ()  [unwired: 12 in]
      }
      event "布尔": Value Change {
        n326 = event-data() -> ("NewVal"=w587:bool)  [unwired: 1 in, 5 out]
        n327 = case shown="False" w587 {
          frame False {
            n328 = global write "VAR总磷总氮全局变量.vi" "权限等级"(enum16{"一级权限", "二级权限", "三级权限", "超级权限"}."一级权限" ("权限等级")) -> ()
          }
          frame True {
            n329 = global read "VAR总磷总氮全局变量.vi" "权限密码"() -> (w591:u32[])
            n330 = global read "VAR总磷总氮全局变量.vi" "权限等级"() -> (w589:enum16{"一级权限", "二级权限", "三级权限", "超级权限"})
            n331 = call "密码权限设置.vi"("权限输入"=w589, "权限密码"=w591) -> ("权限输出"=w590:enum16{"一级权限", "二级权限", "三级权限", "超级权限"})  [unwired: 9 in]
            n332 = global write "VAR总磷总氮全局变量.vi" "权限等级"(w590) -> ()
          }
        }
      }
      event "权限等级": Mouse Down {
        n333 = event-data() -> ()  [unwired: 1 in, 8 out]
        n334 = global read "VAR总磷总氮全局变量.vi" "权限密码"() -> (w594:u32[])
        n335 = global read "VAR总磷总氮全局变量.vi" "权限等级"() -> (w592:enum16{"一级权限", "二级权限", "三级权限", "超级权限"})
        n336 = call "密码权限设置.vi"("权限输入"=w592, "权限密码"=w594) -> ("权限输出"=w593:enum16{"一级权限", "二级权限", "三级权限", "超级权限"})  [unwired: 9 in]
        n337 = global write "VAR总磷总氮全局变量.vi" "权限等级"(w593) -> ()
      }
      event "外设固件": Value Change {
        n338 = event-data() -> ()  [unwired: 1 in, 6 out]
        n339 = call "流程固件设置对话框.vi"() -> ()  [unwired: 12 in]
      }
      event "手动启动": Value Change {
        n340 = event-data() -> ()  [unwired: 1 in, 6 out]
        n341 = call "总磷总氮启动参数对话框.vi"() -> ("确认"=w595:bool, "元素"=w596:cluster{"命令":string, "data":variant})  [unwired: 10 in]
        n342 = case shown="True" w595 {
          tunnel: w597 -> [_ w600]
          tunnel: w596 -> [_ w599]
          frame False {
          }
          frame True {
            n343 = Flush Queue(queue=w600) -> (queue out=w598:refnum<queue>)  [unwired: 1 in, 2 out]
            n344 = Enqueue Element(queue=w598, element=w599) -> ()  [unwired: 2 in, 3 out]
          }
        }
      }
      event "调试": Value Change {
        n345 = event-data() -> ()  [unwired: 1 in, 6 out]
        n346 = call "简易流程调试界面.vi"() -> ()  [unwired: 12 in]
      }
      event "停止": Value Change {
        n347 = event-data() -> ()  [unwired: 1 in, 6 out]
        n348 = Two Button Dialog(message="确认停止？" ("消息")) -> (T button?=w601:bool)  [unwired: 2 in]
        n349 = case shown="True" w601 {
          tunnel: w604 -> [_ w620]
          tunnel: w603 -> [_ w619]
          frame False {
          }
          frame True {
            n350 = Send Notification(notification=TRUE ("通知"), notifier=w619) -> ()  [unwired: 1 in, 2 out]
            n351 = global read "VAR总磷总氮全局变量.vi" "状态告警区"() -> (w614:T4)
            n352 = global read "VAR总磷总氮全局变量.vi" "状态告警区"() -> (w606:T4)
            n353 = Unbundle By Name(w614) -> ("id"=w613:u16)
            n354 = Unbundle By Name(w606) -> ("id"=w605:u16)
            n355 = Bundle By Name(cluster=T17 {"站号"=1, "量程切换"=enum."AUTO", "控制命令"=enum."停止测试", "模式设置"=enum."待机", "测量间隔"=0} ("参数"), "站号"=w613) -> (w615:T17)
            n356 = call "id参数转换.vi"("id"=w605) -> ("table输出"=w607:string)  [unwired: 9 in, 1 out]
            n357 = call "总磷总氮启动命令.vi"("参数"=w615) -> ("启动命令"=w616:cluster{"命令":string, "data":variant})  [unwired: 10 in]
            n358 = Get Date/Time In Seconds() -> (seconds since 1Jan1904=w610:timestamp)
            n359 = Bundle By Name(cluster=T16 {"时间"=timestamp(0 s since 1904-01-01), "参数"="", "日志信息"="", "流程参数"=""} ("data in"), "时间"=w610, "参数"=w607, "日志信息"="手动停止") -> (w611:T16)
            n360 = Enqueue Element(queue=w620, element=w616) -> (error out=w608:errorcluster)  [unwired: 2 in, 2 out]
            n361 = call "总磷总氮操作日志.vi"("错误输入（无错误）"=w608, "data in"=w611) -> ()  [unwired: 9 in, 1 out]
          }
        }
      }
      event "参数设置", "参数查询": Value Change {
        n362 = event-data() -> ()  [unwired: 1 in, 6 out]
        n363 = invoke on="子面板" class="SubPnl" method="Remove VI"() -> (error out=w625:errorcluster)  [unwired: 3 in, 2 out]
        n364 = property on="仪器校准" class="Bool"("Visible"=TRUE ("可见")) -> ()  [unwired: 2 in, 2 out]
        n365 = property on="参数查询" class="Bool"("Visible"=FALSE ("可见")) -> ()  [unwired: 2 in, 2 out]
        n366 = property on="窗格" class="Pane"("Origin"=T3 {"Horizontal"=0, "Vertical"=640} ("原点")) -> ()  [unwired: 2 in, 2 out]
        n367 = invoke on="子面板" class="SubPnl" method="Insert VI"(error in=w625, "VI Ref"=w624) -> ()  [unwired: 2 in, 4 out]
        n368 = global write "VAR总磷总氮全局变量.vi" "页面"(enum16{"主页", "参数页", "校准页"}."参数页" ("页面")) -> ()
      }
      event "仪器校准": Value Change {
        n369 = event-data() -> ()  [unwired: 1 in, 6 out]
        n370 = invoke on="子面板" class="SubPnl" method="Remove VI"() -> (error out=w631:errorcluster)  [unwired: 3 in, 2 out]
        n371 = property on="仪器校准" class="Bool"("Visible"=FALSE ("可见")) -> ()  [unwired: 2 in, 2 out]
        n372 = property on="参数查询" class="Bool"("Visible"=TRUE ("可见")) -> ()  [unwired: 2 in, 2 out]
        n373 = global write "VAR总磷总氮全局变量.vi" "页面"(enum16{"主页", "参数页", "校准页"}."校准页" ("页面")) -> ()
        n374 = invoke on="子面板" class="SubPnl" method="Insert VI"(error in=w631, "VI Ref"=w630) -> ()  [unwired: 2 in, 4 out]
      }
      event "返回": Value Change {
        n375 = event-data() -> ()  [unwired: 1 in, 6 out]
        n376 = global write "VAR总磷总氮全局变量.vi" "页面"(enum16{"主页", "参数页", "校准页"}."主页" ("页面")) -> ()
        n377 = property on="窗格" class="Pane"("Origin"=T3 {"Horizontal"=0, "Vertical"=0} ("原点")) -> ()  [unwired: 2 in, 2 out]
      }
    }
  }
  n378 = while {
    tunnel: w20 -> [w645]
    stop <- FALSE stop-if-true
    n379 = Wait (ms)(milliseconds to wait=u32 1000 ("等待时间（毫秒）")) -> ()  [unwired: 1 out]
    n380 = global read "总磷总氮断电保存全局变量.vi" "MB通信方式选择"() -> (w643:enum16{"串口", "TCP"})
    n381 = global read "VAR总磷总氮全局变量.vi" "升级固件关闭心跳包"() -> (w637:bool)
    n382 = global read "VAR总磷总氮全局变量.vi" "MB session in"() -> (w641:refnum<class "MB_Master.lvclass">)
    n383 = case shown="\"串口\", Default" w643 {
      tunnel: [w648 w649] -> w642
      frame "串口", Default {
        n384 = global read "总磷总氮断电保存全局变量.vi" "VISA Resource"() -> (w648:refnum<visa-resource-name>)
      }
      frame "TCP" {
        n385 = global read "总磷总氮断电保存全局变量.vi" "IP"() -> (w649:string)
      }
    }
    "字符串 2" <- w642
    n386 = property class="MB_Master"(reference=w641) -> ("Properties:Session Valid"=w639:bool)  [unwired: 1 in, 2 out]
    n387 = Not(x=w637) -> (.not. x?=w636:bool)
    n388 = Get Queue Status(queue=w645) -> (queue out=w644:refnum<queue>, # elements in queue=w640:i32)  [unwired: 2 in, 6 out]
    n389 = Equal To 0?(x=w640) -> (x = 0?=w634:bool)
    n390 = Compound Arithmetic op=AND ("复合运算")(w639, w636) -> (w638:bool)
    n391 = global write "VAR总磷总氮全局变量.vi" "心跳包打开状态"(w638) -> ()
    n392 = And(x=w634, y=w638) -> (x .and. y?=w635:bool)
    n393 = case shown="True" w635 {
      tunnel: w644 -> [_ w668]
      frame False {
      }
      frame True {
        n394 = global read "VAR总磷总氮全局变量.vi" "MB session in"() -> (w656:refnum<class "MB_Master.lvclass">)
        n395 = property class="MB_Master"(reference=w656) -> ("Properties:Session Valid"=w654:bool)  [unwired: 1 in, 2 out]
        n396 = global read "VAR总磷总氮全局变量.vi" "通讯状态"() -> (w657:bool)
        n397 = case shown="True" w654 {
          tunnel: [_ w670] -> w653
          frame False {
          }
          frame True {
            n398 = global read "VAR总磷总氮全局变量.vi" "MB session in"() -> (w669:refnum<class "MB_Master.lvclass">)
            n399 = call "版本号读取.vi"("MB session in"=w669) -> ("error out"=w670:errorcluster, "固件版本号"=w671:string)  [unwired: 8 in, 1 out]
            "固件版本号" <- w671
            n400 = global write "VAR总磷总氮全局变量.vi" "固件版本号"(w671) -> ()
          }
        }
        n401 = And(x=w654, y=w657) -> (x .and. y?=w655:bool)
        n402 = case shown="True" w655 {
          tunnel: [_ w672] -> w652
          tunnel: w653 -> [_ w673]
          frame False {
          }
          frame True {
            n403 = global read "VAR总磷总氮全局变量.vi" "MB session in"() -> (w675:refnum<class "MB_Master.lvclass">)
            n404 = call "序列号读取.vi"("Error in"=w673, "MB session in"=w675) -> ("error out"=w672:errorcluster, "序列号"=w674:string)  [unwired: 7 in, 1 out]
            n405 = global write "VAR总磷总氮全局变量.vi" "序列号"(w674) -> ()
          }
        }
        n406 = global read "model config var.vi" "启动队列名称"() -> (w659:cluster{"String":string, "Value":u16}[])
        n407 = for {
          tunnel: [w686] -> w660 mode=indexing
          tunnel: w659 -> [w687] mode=indexing
          tunnel: w652 -> [_]
          n408 = Unbundle By Name(w687) -> ("Value"=w686:u16)
        }
        n409 = for {
          shift-right: [w676] -> w662
          shift-left: w668 -> [w682]
          tunnel: w660 -> [w677] mode=indexing
          n410 = Bundle By Name(cluster=cluster{"命令":string, "data":variant} {"命令"="", "data"=variant} ("元素"), "命令"="读状态告警区", "data"=w677) -> (w684:cluster{"命令":string, "data":variant})
          n411 = Bundle By Name(cluster=cluster{"命令":string, "data":variant} {"命令"="", "data"=variant} ("元素"), "命令"="读测量数据区", "data"=w677) -> (w679:cluster{"命令":string, "data":variant})
          n412 = Enqueue Element(queue=w682, element=w684) -> (queue out=w678:refnum<queue>)  [unwired: 2 in, 2 out]
          n413 = Enqueue Element At Opposite End(queue=w678, element=w679) -> (queue out=w676:refnum<queue>)  [unwired: 2 in, 2 out]
        }
        n414 = global read "VAR总磷总氮全局变量.vi" "状态告警区"() -> (w661:T4)
        n415 = Unbundle By Name(w661) -> ("系统时间"=w650:timestamp)
        n416 = Get Date/Time In Seconds() -> (seconds since 1Jan1904=w667:timestamp)
        n417 = Subtract(x=w667, y=w650) -> (x-y=w666:dbl)
        n418 = Absolute Value(x=w666) -> (abs(x)=w665:dbl)
        n419 = global read "VAR总磷总氮全局变量.vi" "通讯状态"() -> (w651:bool)
        n420 = Greater Or Equal?(x=w665, y=30.0) -> (x >= y?=w663:bool)
        n421 = Compound Arithmetic op=AND ("复合运算")(w663, w651) -> (w658:bool)
        n422 = case shown="True" w658 {
          tunnel: w662 -> [_ w689]
          frame False {
          }
          frame True {
            n423 = call "总磷总氮启动命令.vi"("参数"=T17 {"站号"=3, "量程切换"=enum."AUTO", "控制命令"=enum."校时", "模式设置"=enum."待机", "测量间隔"=0}) -> ("启动命令"=w688:cluster{"命令":string, "data":variant})  [unwired: 10 in]
            n424 = Enqueue Element(queue=w689, element=w688) -> ()  [unwired: 2 in, 3 out]
          }
        }
      }
    }
  }
